vi "UUT Test Info Update and Log.vi"(9 "Where Data":string, 10 "Where Condition":string, 11 "Sequence Context":T1) -> (0 "error out":errorcluster)   [LabVIEW 2023, in "HardwareAbstractionLayer_LVOOP.lvlib" / "Report.lvclass"]
uses:
  Report.lvclass
  <vilib>/addons/TestStand/_TSLegacy.llb/LabVIEW Test - Sequence Context.ctl
  Database/SQL Public VI/Control/DB Options.ctl
  <vilib>/addons/TestStand/_TSUtility.llb/TestStand - Get Property Value (Numeric Array {Signed 16-bit Integer}).vi
  <vilib>/addons/TestStand/_TSUtility.llb/TestStand - Get Property Value (String).vi
  <vilib>/addons/TestStand/_TSUtility.llb/TestStand - Get Property Value (Number {Signed 32-bit Integer}).vi
  Database/Database.lvclass
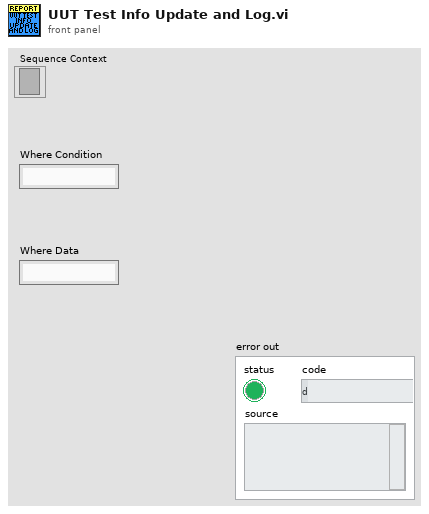
[diagram p1: front panel]
types:
  T1 = typedef "LabVIEW Test - Sequence Context.ctl" = refnum<k7>
  T2 = typedef "HardwareAbstractionLayer_LVOOP.lvlib/Database.lvclass/DB Options.ctl" = enum16{"Init", "Select Data", "Insert Data", "Update Data", "Delete Data", "Execute Query", "Create Schema", "Create Table", "List Tables", "List Columns", "Close"}
  T3 = typedef "HardwareAbstractionLayer_LVOOP.lvlib/Report.lvclass/Result FGV Data.ctl" = cluster{"Project Name":string, "Product Name":string, "Product Varient":string, "Test Name":string, "Test Phase":string, "Test Description":string, "Temp Chamber Name":string, "Schema":string, "Total No of Cycles":u32, "Current Cycle Number":u32, "Cycle Duration":u32, "Current Test Mode":string}
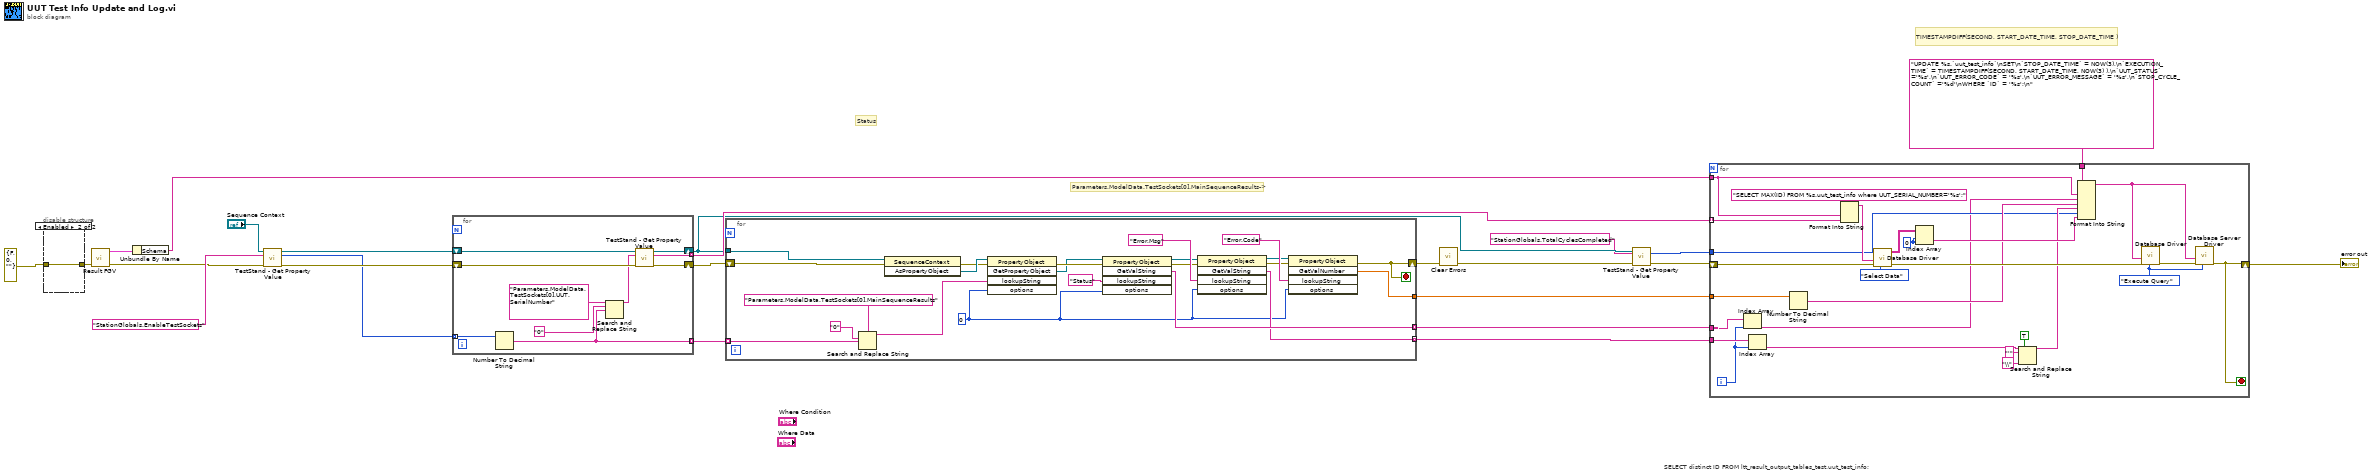
[diagram p0: block diagram]
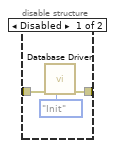
[diagram p2: hidden frame]
diagram:
  # "Parameters.ModelData.TestSockets[0].MainSequenceResults->"
  # "TIMESTAMPDIFF(SECOND, START_DATE_TIME, STOP_DATE_TIME )"
  # "Status"
  # "SELECT distinct ID FROM ltt_result_output_tables_test.uut_test_info;"
  n1 = disable-structure shown="Enabled" {
    disable-tunnel: errorcluster {"status"=FALSE, "code"=0, "source"=""} ("error in") -> [w26 w28]
    disable-tunnel: [w25 w28] -> w14
    frame Disabled {
      n2 = call "Database Driver.vi"("Options"=DB_Options."Init", "error in"=w26) -> ("error out"=w25:errorcluster)  [unwired: 6 in, 3 out]
    }
    frame Enabled {
    }
  }
  n3 = call "Result FGV.vi"("error in"=w14) -> ("error out"=w20:errorcluster, "Result FGV Data Out"=w24:T3)  [unwired: 9 in]
  n4 = Unbundle By Name(w24) -> ("Schema"=w16:string)
  n5 = call-poly <vilib>:"TestStand - Get Property Value.vi"("Sequence Context In"="Sequence Context", "Lookup String"="StationGlobals.EnableTestSockets", "error in (no error)"=w20) -> ("Sequence Context Out"=w23:refnum<k7>, "Value"=w3:i16[], "error out"=w19:errorcluster)  [unwired: 10 in]
  n6 = for {
    tunnel: [w36] -> w18 mode=indexing
    tunnel: w3 -> [w34] mode=indexing
    tunnel: [w30] -> w2 mode=indexing
    shift-right: [w35] -> w11
    shift-left: w23 -> [w38]
    shift-right: [w29] -> w1
    shift-left: w19 -> [w37]
    n7 = Number To Decimal String(number=w34) -> (decimal integer string=w30:string)  [unwired: 1 in]
    n8 = Search and Replace String(input string="Parameters.ModelData.TestSockets[0].UUT.SerialNumber" ("Lookup String"), search string="0", replace string=w30) -> (result string=w31:string)  [unwired: 5 in, 3 out]
    n9 = call-poly <vilib>:"TestStand - Get Property Value.vi"("Sequence Context In"=w38, "Lookup String"=w31, "error in (no error)"=w37) -> ("Sequence Context Out"=w35:refnum<k7>, "Value"=w36:string, "error out"=w29:errorcluster)  [unwired: 10 in]
  }
  n10 = for {
    tunnel: [w60] -> w17 mode=indexing
    tunnel: [w59] -> w13
    tunnel: [w58] -> w12 mode=indexing
    tunnel: w11 -> [w57]
    tunnel: w2 -> [w55] mode=indexing
    shift-right: [w39] -> w10
    shift-left: w1 -> [w50]
    stop <- w39 stop-if-true
    w45 = 0 ("options")
    n11 = Search and Replace String(input string="Parameters.ModelData.TestSockets[0].MainSequenceResults" ("Lookup String"), search string="0", replace string=w55) -> (result string=w52:string)  [unwired: 5 in, 3 out]
    n12 = invoke class="SequenceContext" method="AsPropertyObject"(reference=w57, error in=w50) -> (error out=w49:errorcluster, "AsPropertyObject"=w53:refnum<k7>)  [unwired: 1 in, 1 out]
    n13 = invoke class="PropertyObject" method="GetPropertyObject"(reference=w53, error in=w49, "lookupString"=w52, "options"=w45) -> (error out=w48:errorcluster, "GetPropertyObject"=w40:refnum<k7>)  [unwired: 1 in, 3 out]
    n14 = invoke class="PropertyObject" method="GetValString"(reference=w40, error in=w48, "lookupString"="Status", "options"=w45) -> (reference out=w44:refnum<k7>, error out=w42:errorcluster, "GetValString"=w60:string)  [unwired: 1 in, 2 out]
    n15 = invoke class="PropertyObject" method="GetValString"(reference=w44, error in=w42, "lookupString"="Error.Msg", "options"=w45) -> (reference out=w43:refnum<k7>, error out=w41:errorcluster, "GetValString"=w58:string)  [unwired: 1 in, 2 out]
    n16 = invoke class="PropertyObject" method="GetValNumber"(reference=w43, error in=w41, "lookupString"="Error.Code", "options"=w45) -> (error out=w39:errorcluster, "GetValNumber"=w59:dbl)  [unwired: 1 in, 3 out]
  }
  n17 = call <vilib>:"Clear Errors.vi"("error in (no error)"=w10) -> ("error out"=w8:errorcluster)  [unwired: 5 in, 1 out]
  n18 = call-poly <vilib>:"TestStand - Get Property Value.vi"("Sequence Context In"=w11, "Lookup String"="StationGlobals.TotalCyclesCompleted", "error in (no error)"=w8) -> ("Value"=w4:i32, "error out"=w6:errorcluster)  [unwired: 10 in, 1 out]
  n19 = for {
    tunnel: w16 -> [w78]
    shift-right: [w63] -> w9
    shift-left: w6 -> [w85]
    tunnel: w18 -> [w70] mode=indexing
    tunnel: w17 -> [w69]
    tunnel: w13 -> [w81]
    tunnel: w12 -> [w68]
    tunnel: "UPDATE %s.`uut_test_info`\nSET\n`STOP_DATE_TIME` = NOW(3),\n`EXECUTION_TIME` = TIMESTAMPDIFF(SECOND, START_DATE_TIME, NOW(3) ),\n`UUT_STATUS` ='%s',\n`UUT_ERROR_CODE` = '%s',\n`UUT_ERROR_MESSAGE` = '%s',\n`STOP_CYCLE_COUNT` ='%d'\nWHERE `ID` = '%s';\n" ("format string") -> [w79]
    tunnel: w4 -> [w71]
    i -> [w67]
    stop <- w63 stop-if-true
    w62 = DB_Options."Execute Query" ("Options")
    w72 = 0 ("disabled index (col)")
    n20 = Index Array(array=w69, index=w67) -> (element=w65:string)
    n21 = Index Array(array=w68, index=w67) -> (element=w66:string)
    n22 = Number To Decimal String(number=w81) -> (decimal integer string=w77:string)  [unwired: 1 in]
    n23 = Format Into String(format string="SELECT MAX(ID) FROM %s.uut_test_info where UUT_SERIAL_NUMBER='%s';", w78, w70) -> (resulting string=w86:string)  [unwired: 2 in, 1 out]
    n24 = call "Database Driver.vi"("Options"=DB_Options."Select Data", "error in"=w85, "SQL query"=w86) -> ("error out"=w80:errorcluster, "data"=w84:string[][])  [unwired: 5 in, 2 out]
    n25 = Index Array(array=w84, index (row)=w72, index (col)=w72) -> (element=w83:string)
    n26 = Search and Replace String(replace all?=TRUE ("replace all? (F)"), input string=w66, search string="'", replace string="\\" ("replace string (\"\")")) -> (result string=w76:string)  [unwired: 4 in, 3 out]
    n27 = Format Into String(format string=w79, w78, w65, w77, w76, w71, w83) -> (resulting string=w61:string)  [unwired: 2 in, 1 out]
    n28 = call "Database Driver.vi"("Options"=w62, "error in"=w80, "SQL query"=w61) -> ("error out"=w64:errorcluster)  [unwired: 5 in, 3 out]
    n29 = call "Database Server Driver.vi"("Options"=w62, "error in"=w64, "SQL query"=w61) -> ("error out"=w63:errorcluster)  [unwired: 5 in, 3 out]
  }
  "error out" <- w9
